vi "Play Log.vi"(9 "file path":path=path "c:/test", 11 "rt fifo":refnum<k33>) -> ()   [LabVIEW 2013]
uses:
  dashboard/TeleopCmd.ctl
  CmdFlag.ctl
panel:
  out "x = y?":bool
  out "file or folder exists?":bool
  out "x-y":dbl
  out "element 2":dbl
  out "element":dbl
  out "error out":errorcluster
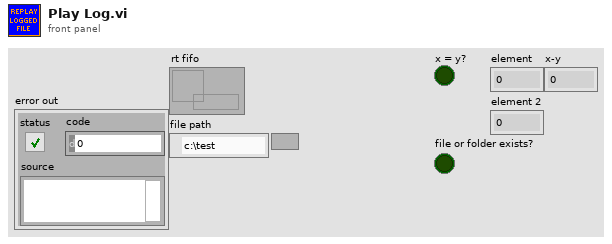
[diagram p1: front panel]
types:
  T1 = typedef "TeleopCmd.ctl" = cluster{"Left Joystick":dbl, "Right Joystick":dbl, "Shift":bool, "CmdFlag":T2}
  T2 = typedef "CmdFlag.ctl" = enum16{"noop", "suspend", "resume"}
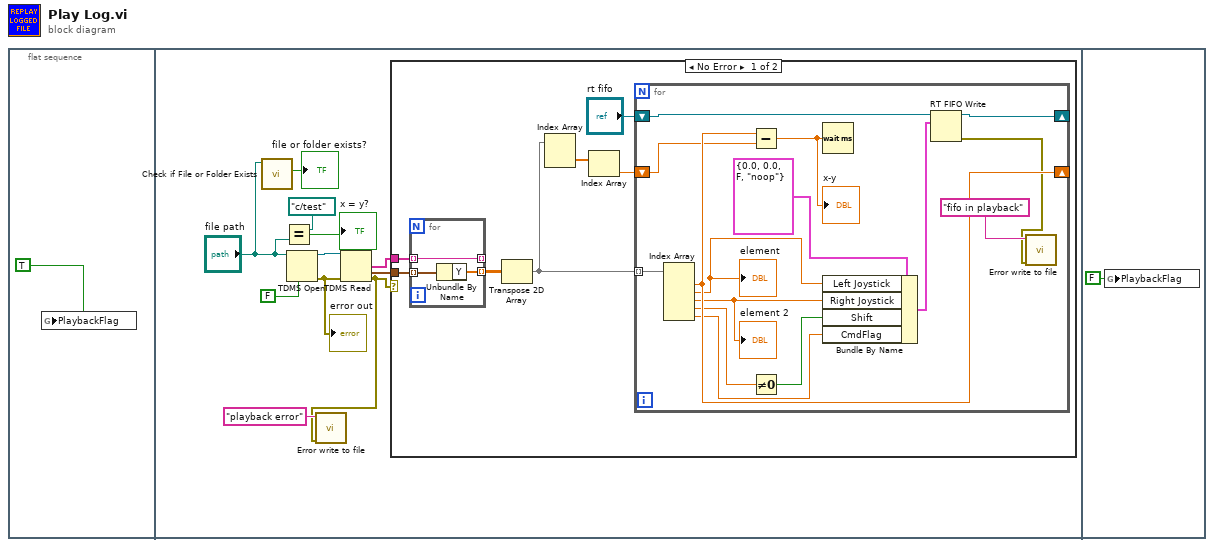
[diagram p0: block diagram]
diagram:
  n1 = flat-sequence {
    frame #0 {
      n2 = global write "PlaybackOn" "PlaybackFlag"(TRUE ("PlaybackFlag")) -> ()
    }
    frame #1 {
      n3 = call <vilib>:"Check if File or Folder Exists.vi"("path"="file path") -> ("file or folder exists?"=→"file or folder exists?":bool)  [unwired: 8 in, 2 out]
      n4 = Equal?(x=path "c:/test" ("file path"), y="file path") -> (x = y?=→"x = y?":bool)
      n5 = TDMS Open(6:FALSE ("disable buffering? (T)"), 11:"file path") -> (0:w8:errorcluster, 3:w11:refnum<k34>)  [unwired: 5 in]
      "error out" <- w8
      n6 = TDMS Read(0:w11, 11:w8) -> (8:w10:string[], 10:w9:waveform(dbl)[], 15:w2:errorcluster)  [unwired: 6 in, 3 out]
      n7 = call "Error write to file.vi"("error in (no error)"=w2, "Description"="playback error") -> ()  [unwired: 10 in]
      n8 = case shown="No Error" w2 {
        tunnel: w10 -> [w19 _]
        tunnel: w9 -> [w18 _]
        frame No Error {
          n9 = for {
            tunnel: w19 -> [w35] mode=indexing
            tunnel: w18 -> [w37] mode=indexing
            tunnel: [w36] -> w17 mode=indexing
            tunnel: [w35] -> _ mode=indexing
            n10 = Unbundle By Name(w37) -> ("Y"=w36:dbl[])
          }
          n11 = Transpose 2D Array(2D array=w17) -> (transposed array=w16:dbl[][])
          n12 = Index Array(array=w16) -> (element=w15:dbl[])  [unwired: 2 in]
          n13 = Index Array(array=w15) -> (element=w14:dbl)  [unwired: 1 in]
          n14 = for {
            tunnel: w16 -> [w34] mode=indexing
            shift-right: [w33] -> _
            shift-left: w14 -> [w32]
            shift-right: [w23] -> _
            shift-left: "rt fifo" -> [w22]
            n15 = Index Array(array=w34) -> (element #1=w33:dbl, element #2=w28:dbl, element #3=w29:dbl, element #4=w27:dbl, element #5=w25:dbl)  [unwired: 5 in]
            "element" <- w28
            "element 2" <- w29
            n16 = Subtract(x=w33, y=w32) -> (x-y=w31:dbl)
            "x-y" <- w31
            n17 = Not Equal To 0?(x=w27) -> (x != 0?=w26:bool)
            n18 = Wait (ms)(milliseconds to wait=w31) -> ()  [unwired: 1 out]
            n19 = Bundle By Name(cluster=T1 {"Left Joystick"=0.0, "Right Joystick"=0.0, "Shift"=FALSE, "CmdFlag"=enum."noop"} ("Cluster"), "Left Joystick"=w28, "Right Joystick"=w29, "Shift"=w26, "CmdFlag"=w25) -> (w24:T1)
            n20 = RT FIFO Write(0:w22, 1:w24) -> (8:w23:refnum<k33>, 11:w20:errorcluster)  [unwired: 3 in, 2 out]
            n21 = call "Error write to file.vi"("error in (no error)"=w20, "Description"="fifo in playback") -> ()  [unwired: 10 in]
          }
        }
        frame Error {
        }
      }
    }
    frame #2 {
      n22 = global write "PlaybackOn" "PlaybackFlag"(FALSE ("PlaybackFlag")) -> ()
    }
  }
